vi "mecanum_begin.vi"   [LabVIEW 2012]
uses:
  <vilib>/Rock Robotics/WPI/CAN/Jaguar/SubVIs/WPI_CANJaguar_ControlMode.ctl
  <vilib>/Rock Robotics/WPI/CAN/Jaguar/SubVIs/WPI_CANJaguar_BrakeCoastMode.ctl
  <vilib>/Rock Robotics/WPI/CAN/Jaguar/SubVIs/WPI_CANJaguar_SpeedReference.ctl
  <vilib>/Rock Robotics/WPI/MotorControl/WPI_MotorControlOpenCANJaguar.vi
types:
  T1 = typedef "WPI_CANJaguar_SpeedReference.ctl" = u8
  T2 = typedef "WPI_CANJaguar_BrakeCoastMode.ctl" = enum8{"Jumper", "Brake", "Coast"}
  T3 = typedef "WPI_CANJaguar_ControlMode.ctl" = enum8{"Percent VBus", "Current", "Speed", "Position", "Voltage"}
  T4 = typedef "WPI_MotorControlDeviceRef.ctl" = cluster{"DeviceStatus":errorcluster, "Type":enum16{"PWM", "CAN"}, "PWM":cluster{"Digital Module":T5, "PWM Channel":T6, "DeadBand":T7}, "CAN":cluster{"Device Number":u8, "Control Mode":T3, "Semaphore":T8, "Max Vout":dbl}, "Invert":bool, "TransformRef":T9, "InvTransformRef":T9}
  T5 = typedef "FPGA_TypedefDigitalModule.ctl" = enum16{"Digital Module 1", "Digital Module 2"}
  T6 = typedef "FPGA_DIOPWMChannel.ctl" = enum8{"PWM 1", "PWM 2", "PWM 3", "PWM 4", "PWM 5", "PWM 6", "PWM 7", "PWM 8", "PWM 9", "PWM 10", "Invalid"}
  T7 = typedef "WPI_PWMDeadband.ctl" = cluster{"Name":string, "maxPositivePwm":i32, "minPositivePwm":i32, "centerPwm":i32, "maxNegativePwm":i32, "minNegativePwm":i32, "angularRange":u16}
  T8 = typedef "Semaphore RefNum" = refnum<k1>
  T9 = typedef "WPI_PWMTransform_ConPane.ctl" = refnum<vi>
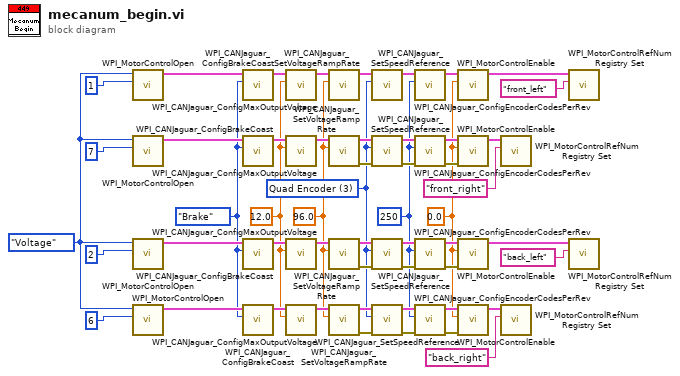
[diagram p0: block diagram]
diagram:
  w1 = T1 3 items=["Encoder"=0, "Inv Encoder"=2, "Quad Encoder"=3, "None"=255] ("Speed Reference")
  w2 = 0.0 ("Encoder Initial Position")
  w3 = u16 250 ("Encoder Codes Per Rev")
  w25 = 96.0 ("VoltageRampRate (V/s)")
  w30 = 12.0 ("Maximum Output Voltage")
  w35 = WPI_CANJaguar_BrakeCoastMode."Brake" ("Brake / Coast Mode")
  w36 = WPI_CANJaguar_ControlMode."Voltage" ("Control Mode")
  n1 = call-poly <vilib>:"WPI_MotorControlOpen.vi"("Device Number"=u8 1, "Control Mode"=w36) -> ("MotorControlDeviceRef"=w52:T4)  [unwired: 8 in, 1 out]
  n2 = call-poly <vilib>:"WPI_MotorControlOpen.vi"("Device Number"=u8 7, "Control Mode"=w36) -> ("MotorControlDeviceRef"=w43:T4)  [unwired: 8 in, 1 out]
  n3 = call-poly <vilib>:"WPI_MotorControlOpen.vi"("Device Number"=u8 2, "Control Mode"=w36) -> ("MotorControlDeviceRef"=w49:T4)  [unwired: 8 in, 1 out]
  n4 = call-poly <vilib>:"WPI_MotorControlOpen.vi"("Device Number"=u8 6, "Control Mode"=w36) -> ("MotorControlDeviceRef"=w46:T4)  [unwired: 8 in, 1 out]
  n5 = call <vilib>:"WPI_CANJaguar_ConfigBrakeCoast.vi"("Brake / Coast Mode"=w35, "CAN Jaguar Ref"=w52) -> ("CAN Jaguar Ref Out"=w34:T4)  [unwired: 8 in, 1 out]
  n6 = call <vilib>:"WPI_CANJaguar_ConfigBrakeCoast.vi"("Brake / Coast Mode"=w35, "CAN Jaguar Ref"=w43) -> ("CAN Jaguar Ref Out"=w31:T4)  [unwired: 8 in, 1 out]
  n7 = call <vilib>:"WPI_CANJaguar_ConfigBrakeCoast.vi"("Brake / Coast Mode"=w35, "CAN Jaguar Ref"=w49) -> ("CAN Jaguar Ref Out"=w33:T4)  [unwired: 8 in, 1 out]
  n8 = call <vilib>:"WPI_CANJaguar_ConfigBrakeCoast.vi"("Brake / Coast Mode"=w35, "CAN Jaguar Ref"=w46) -> ("CAN Jaguar Ref Out"=w32:T4)  [unwired: 8 in, 1 out]
  n9 = call <vilib>:"WPI_CANJaguar_ConfigMaxOutputVoltage.vi"("Maximum Output Voltage"=w30, "CAN Jaguar Ref"=w34) -> ("CAN Jaguar Ref Out"=w26:T4)  [unwired: 8 in, 1 out]
  n10 = call <vilib>:"WPI_CANJaguar_ConfigMaxOutputVoltage.vi"("Maximum Output Voltage"=w30, "CAN Jaguar Ref"=w31) -> ("CAN Jaguar Ref Out"=w29:T4)  [unwired: 8 in, 1 out]
  n11 = call <vilib>:"WPI_CANJaguar_ConfigMaxOutputVoltage.vi"("Maximum Output Voltage"=w30, "CAN Jaguar Ref"=w33) -> ("CAN Jaguar Ref Out"=w27:T4)  [unwired: 8 in, 1 out]
  n12 = call <vilib>:"WPI_CANJaguar_ConfigMaxOutputVoltage.vi"("Maximum Output Voltage"=w30, "CAN Jaguar Ref"=w32) -> ("CAN Jaguar Ref Out"=w28:T4)  [unwired: 8 in, 1 out]
  n13 = call <vilib>:"WPI_CANJaguar_SetVoltageRampRate.vi"("VoltageRampRate (V/s)"=w25, "CAN Jaguar Ref"=w26) -> ("CAN Jaguar Ref Out"=w24:T4)  [unwired: 8 in, 1 out]
  n14 = call <vilib>:"WPI_CANJaguar_SetVoltageRampRate.vi"("VoltageRampRate (V/s)"=w25, "CAN Jaguar Ref"=w29) -> ("error out"=w13:errorcluster, "CAN Jaguar Ref Out"=w12:T4)  [unwired: 8 in]
  n15 = call <vilib>:"WPI_CANJaguar_SetVoltageRampRate.vi"("VoltageRampRate (V/s)"=w25, "CAN Jaguar Ref"=w27) -> ("error out"=w6:errorcluster, "CAN Jaguar Ref Out"=w7:T4)  [unwired: 8 in]
  n16 = call <vilib>:"WPI_CANJaguar_SetVoltageRampRate.vi"("VoltageRampRate (V/s)"=w25, "CAN Jaguar Ref"=w28) -> ("error out"=w19:errorcluster, "CAN Jaguar Ref Out"=w18:T4)  [unwired: 8 in]
  n17 = call <vilib>:"WPI_CANJaguar_SetSpeedReference.vi"("Speed Reference"=w1, "CAN Jaguar Ref"=w24) -> ("CAN Jaguar Ref Out"=w23:T4)  [unwired: 8 in, 1 out]
  n18 = call <vilib>:"WPI_CANJaguar_SetSpeedReference.vi"("error in (no error)"=w13, "Speed Reference"=w1, "CAN Jaguar Ref"=w12) -> ("error out"=w11:errorcluster, "CAN Jaguar Ref Out"=w10:T4)  [unwired: 7 in]
  n19 = call <vilib>:"WPI_CANJaguar_SetSpeedReference.vi"("error in (no error)"=w6, "Speed Reference"=w1, "CAN Jaguar Ref"=w7) -> ("error out"=w4:errorcluster, "CAN Jaguar Ref Out"=w5:T4)  [unwired: 7 in]
  n20 = call <vilib>:"WPI_CANJaguar_SetSpeedReference.vi"("error in (no error)"=w19, "Speed Reference"=w1, "CAN Jaguar Ref"=w18) -> ("error out"=w17:errorcluster, "CAN Jaguar Ref Out"=w16:T4)  [unwired: 7 in]
  n21 = call <vilib>:"WPI_CANJaguar_ConfigEncoderCodesPerRev.vi"("Encoder Codes Per Rev"=w3, "CAN Jaguar Ref"=w23) -> ("CAN Jaguar Ref Out"=w22:T4)  [unwired: 8 in, 1 out]
  n22 = call <vilib>:"WPI_CANJaguar_ConfigEncoderCodesPerRev.vi"("error in (no error)"=w11, "Encoder Codes Per Rev"=w3, "CAN Jaguar Ref"=w10) -> ("error out"=w8:errorcluster, "CAN Jaguar Ref Out"=w9:T4)  [unwired: 7 in]
  n23 = call <vilib>:"WPI_CANJaguar_ConfigEncoderCodesPerRev.vi"("error in (no error)"=w4, "Encoder Codes Per Rev"=w3, "CAN Jaguar Ref"=w5) -> ("error out"=w20:errorcluster, "CAN Jaguar Ref Out"=w21:T4)  [unwired: 7 in]
  n24 = call <vilib>:"WPI_CANJaguar_ConfigEncoderCodesPerRev.vi"("error in (no error)"=w17, "Encoder Codes Per Rev"=w3, "CAN Jaguar Ref"=w16) -> ("error out"=w14:errorcluster, "CAN Jaguar Ref Out"=w15:T4)  [unwired: 7 in]
  n25 = call <vilib>:"WPI_MotorControlEnable.vi"("Encoder Initial Position"=w2, "CAN Jaguar Ref"=w22) -> ("CAN Jaguar Ref Out"=w51:T4)  [unwired: 8 in, 1 out]
  n26 = call <vilib>:"WPI_MotorControlEnable.vi"("error in (no error)"=w8, "Encoder Initial Position"=w2, "CAN Jaguar Ref"=w9) -> ("CAN Jaguar Ref Out"=w42:T4)  [unwired: 7 in, 1 out]
  n27 = call <vilib>:"WPI_MotorControlEnable.vi"("error in (no error)"=w20, "Encoder Initial Position"=w2, "CAN Jaguar Ref"=w21) -> ("CAN Jaguar Ref Out"=w48:T4)  [unwired: 7 in, 1 out]
  n28 = call <vilib>:"WPI_MotorControlEnable.vi"("error in (no error)"=w14, "Encoder Initial Position"=w2, "CAN Jaguar Ref"=w15) -> ("CAN Jaguar Ref Out"=w45:T4)  [unwired: 7 in, 1 out]
  n29 = call <vilib>:"WPI_MotorControlRefNum Registry Set.vi"("refnum name"="front_right", "MotorControlDevRef"=w42) -> ()  [unwired: 8 in, 2 out]
  n30 = call <vilib>:"WPI_MotorControlRefNum Registry Set.vi"("refnum name"="back_right", "MotorControlDevRef"=w45) -> ()  [unwired: 8 in, 2 out]
  n31 = call <vilib>:"WPI_MotorControlRefNum Registry Set.vi"("refnum name"="front_left", "MotorControlDevRef"=w51) -> ()  [unwired: 8 in, 2 out]
  n32 = call <vilib>:"WPI_MotorControlRefNum Registry Set.vi"("refnum name"="back_left", "MotorControlDevRef"=w48) -> ()  [unwired: 8 in, 2 out]
